vi "实验第四题.vi"() -> ()   [LabVIEW 2018]
panel:
  in  "温度上限（摄氏）":dbl
  in  "stop 2":bool
  in  "暂停":bool
  in  "暂停采集":bool
  in  "显示模式":bool
  out "采集进度":u8(slide) scale=0.0..100.0
  out "温度计":dbl(slide) scale=0.0..100.0
  out "Alarm Counter":dbl
  in  "开始":bool
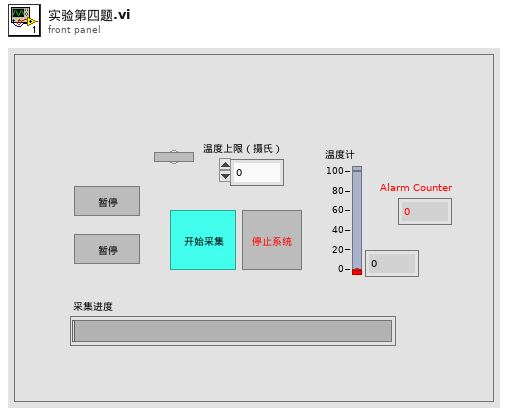
[diagram p1: front panel]
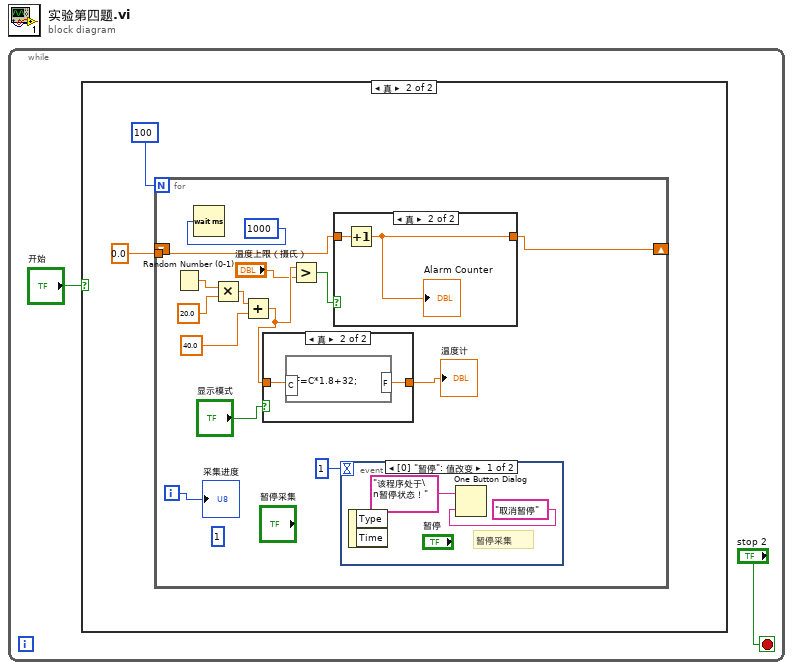
[diagram p0: block diagram]
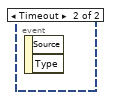
[diagram p3: hidden frame]
diagram:
  n1 = while {
    stop <- "stop 2" stop-if-true
    n2 = case shown="真" "开始" {
      frame False {
      }
      frame True {
        n3 = for {
          N: u32 100 ("milliseconds to wait") -> [_]
          tunnel: 0.0 -> [w18]
          shift-right: [w8] -> _
          shift-left: _ -> [_]
          i -> [w12]
          (unwired) u32 1 ("milliseconds to wait")
          n4 = Random Number (0-1)() -> (number: 0 to 1=w16:dbl)
          n5 = Wait (ms)(milliseconds to wait=u32 1000) -> ()  [unwired: 1 out]
          n6 = Multiply(x=w16, y=20.0) -> (x*y=w14:dbl)
          n7 = Add(x=w14, y=40.0) -> (x+y=w6:dbl)
          n8 = case shown="真" "显示模式" {
            tunnel: w6 -> [w21 w23]
            tunnel: [w21 w22] -> w11
            frame False {
            }
            frame True {
              n9 = formula code="F=C*1.8+32;"("C"=w23) -> ("F"=w22:dbl)
            }
          }
          "温度计" <- w11
          n10 = Greater?(x=w6, y="温度上限（摄氏）") -> (0:w7:bool)
          n11 = case shown="真" w7 {
            tunnel: [w24 w26] -> w8
            tunnel: w18 -> [w24 w25]
            frame False {
            }
            frame True {
              n12 = Increment(x=w25) -> (x+1=w26:dbl)
              "Alarm Counter" <- w26
            }
          }
          n13 = event shown="[0] \"暂停\": 值改变" {
            selector: _ -> [_ _]
            dyn-events: _ -> [_ _]
            timeout: 1 -> [_ _]
            event "暂停": Value Change {
              # "暂停采集"
              n14 = event-data() -> ()  [unwired: 1 in, 2 out]
              n15 = One Button Dialog(message="该程序处于\n暂停状态！", button name ("OK")="取消暂停" ("message")) -> ()  [unwired: 1 out]
            }
            event Timeout {
              n16 = event-data() -> ()  [unwired: 1 in, 2 out]
            }
          }
          "采集进度" <- w12
        }
      }
    }
  }
